vi "MainVI.vi"() -> ()   [LabVIEW 2020]
doc: "Main VI for Local Server on RPi and communication with cliend."
uses:
  <vilib>/MakerHub/LINX/Private/Type Defs/Peripherals/SPI/SPI Configuration.ctl
  <vilib>/MakerHub/LINX/Private/Type Defs/Peripherals/SPI/SPI Bit Order.ctl
  <vilib>/MakerHub/LINX/Private/Type Defs/Peripherals/SPI/SPI Mode.ctl
  Custom Ctls/Akcija.ctl
  Custom Ctls/States.ctl
  <vilib>/MediaMongrels Ltd/WebSockets/Sockets/VISA TCP Listener/VISA TCP Listener.lvclass
  <vilib>/MediaMongrels Ltd/WebSockets/WebSockets/WebSocket/WebSocket.lvclass
  <vilib>/MakerHub/LINX/Public/Peripherals/SPI/SPI CS Config.ctl
  <vilib>/MakerHub/LINX/Private/Type Defs/Peripherals/SPI/SPI CS Logic Level.ctl
  <vilib>/MediaMongrels Ltd/WebSockets/WebSockets/WebSocket Server/WebSocket Server.lvclass
  C:/Program Files (x86)/National Instruments/LabVIEW 2020/vi.lib/MediaMongrels Ltd/WebSockets/WebSockets/WebSocket/WebSocket.lvclass
  <vilib>/MakerHub/LINX/Public/Peripherals/SPI/SPI Write Read 1 Frame.vi
  <vilib>/MakerHub/LINX/Public/Peripherals/SPI/SPI Write Read N Frames.vi
  <vilib>/MakerHub/LINX/Private/Local IO/LinxSpiWriteRead.vi
  <vilib>/MakerHub/LINX/Public/Utilities/Check Channel.vi
  <vilib>/MakerHub/LINX/Private/Local IO/Handle Errors.vi
  <vilib>/MakerHub/LINX/Public/Utilities/Open Local.vi
  <vilib>/MakerHub/LINX/Private/Utilties/Generate Error.vi
  <vilib>/MakerHub/LINX/LMH-LINX.lvlib
panel:
  in  "Stop":bool
  out "String":string
  in  "Client Closed":string="The client VI closed the connection."
  in  "SPI Configuration":T1={"Clock Frequency"=1000000, "Bit Order"=enum."MSb First", "SPI Mode"=enum."Mode 0"}
  out "Output":u8[](array[numeric])
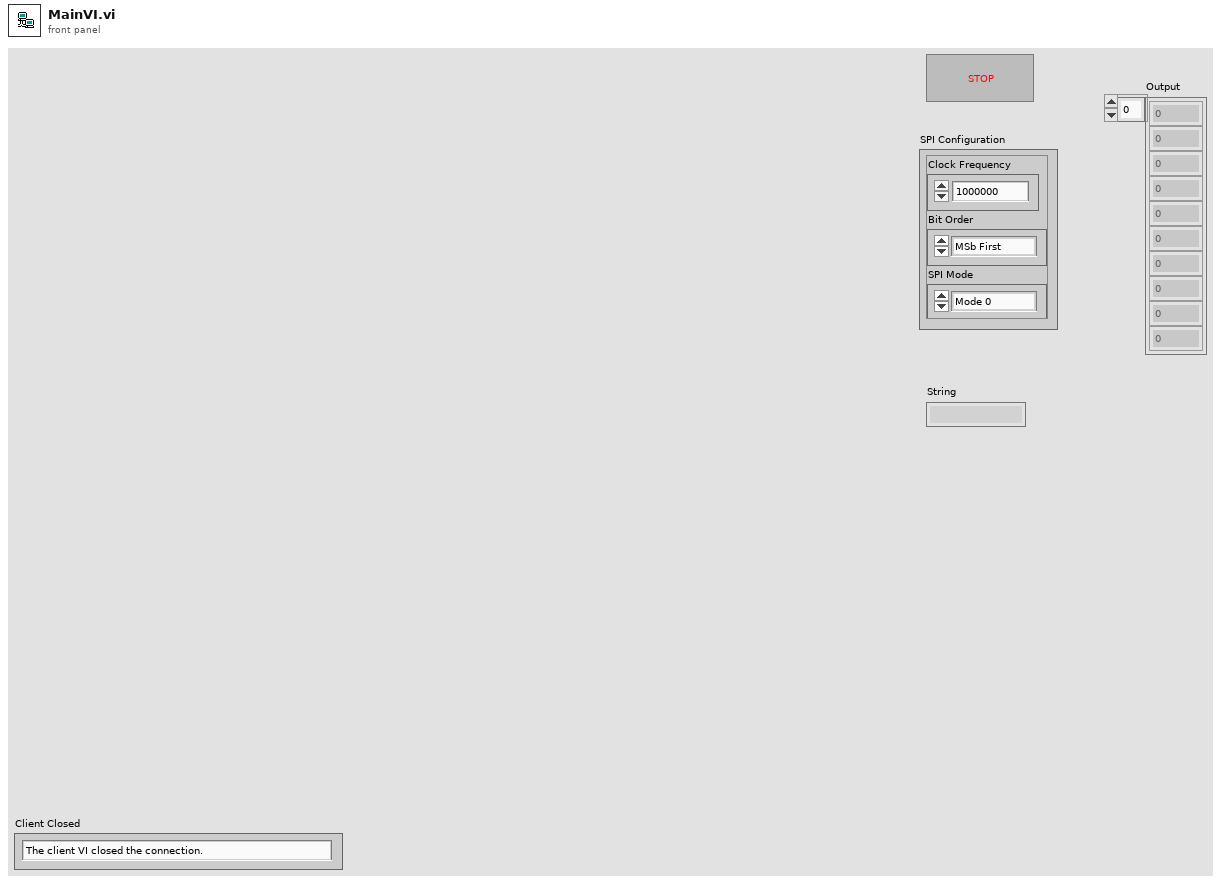
[diagram p1: front panel]
types:
  T1 = typedef "LMH-LINX.lvlib/SPI Configuration.ctl" = cluster{"Clock Frequency":u32, "Bit Order":T2, "SPI Mode":T3}
  T2 = typedef "LMH-LINX.lvlib/SPI Bit Order.ctl" = enum8{"LSb First", "MSb First"}
  T3 = typedef "LMH-LINX.lvlib/SPI Mode.ctl" = enum8{"Mode 0", "Mode 1", "Mode 2", "Mode 3"}
  T4 = typedef "States.ctl" = enum16{"Initialise", "Listen", "Read Data", "Close WebSocket", "Exit"}
  T5 = typedef "Akcija.ctl" = enum16{"Initialize", "Write", "Read", "Update"}
  T6 = typedef "LMH-LINX.lvlib/LINX Ref.ctl" = cluster{"IO":T7, "Interface":T8, "LINX Device Config":T9}
  T7 = typedef "LMH-LINX.lvlib/Platform.ctl" = enum16{"Remote", "Local"}
  T8 = typedef "LMH-LINX.lvlib/Interface.ctl" = enum16{"Serial", "TCP"}
  T9 = typedef "LMH-LINX.lvlib/Device.lvlib/LINX Device Config.ctl" = cluster{"Interface":T8, "COM Port":refnum<visa-resource-name>, "TCP Configuration":T10, "Device Family":u8, "Device ID":u8, "Device Name":string, "TCP Ref":refnum<k5>, "Channels":T11}
  T10 = typedef "LMH-LINX.lvlib/Device.lvlib/TCP Config.ctl" = cluster{"IP Address":string, "Port":u16}
  T11 = typedef "LMH-LINX.lvlib/Channels.ctl" = cluster{"DI":u8[], "DO":u8[], "AI":u8[], "AO":u8[], "PWM":u8[], "QE":u8[], "UART":u8[], "I2C 2":u8[], "SPI":u8[], "CAN":u8[], "Servo":u8[], "AI Ref (V)":dbl, "AI Resolution (Bits)":u8, "AO Ref (V)":dbl, "AO Resolution (Bits)":u8}
  T12 = typedef "LMH-LINX.lvlib/SPI CS Config.ctl" = cluster{"CS Channel":u8, "CS Logic Level":T13}
  T13 = typedef "LMH-LINX.lvlib/SPI CS Logic Level.ctl" = enum8{"Active Low", "Active High"}
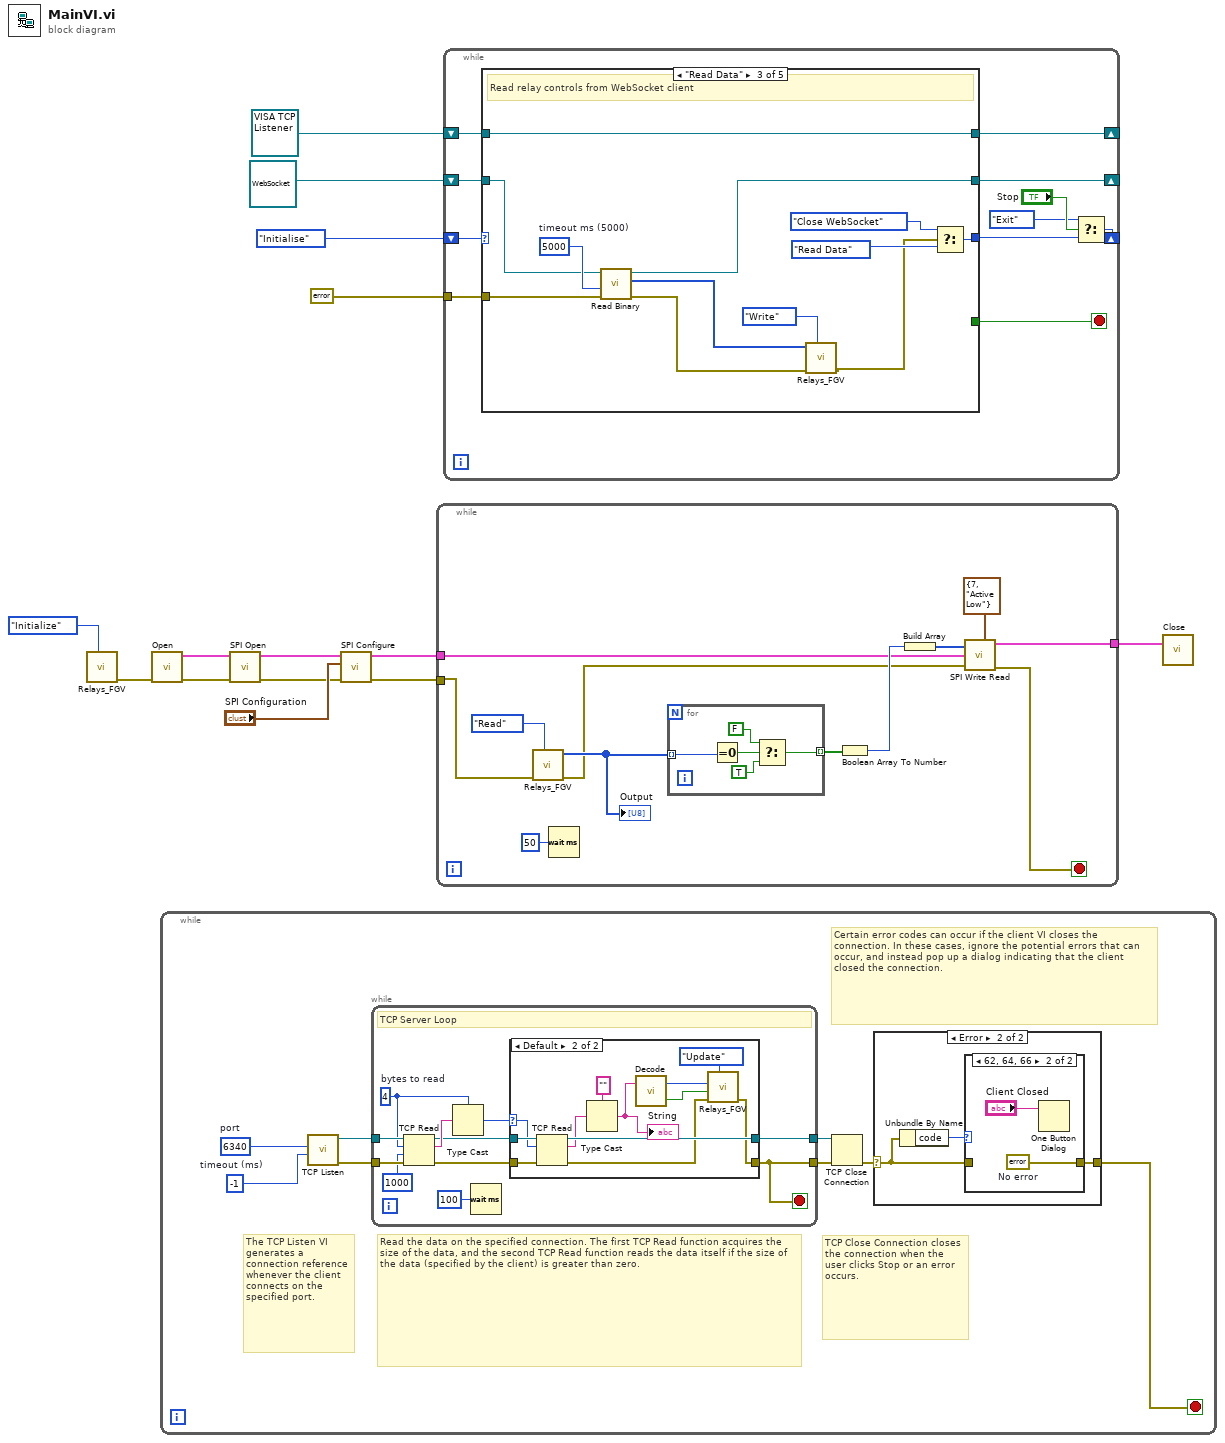
[diagram p0: block diagram]
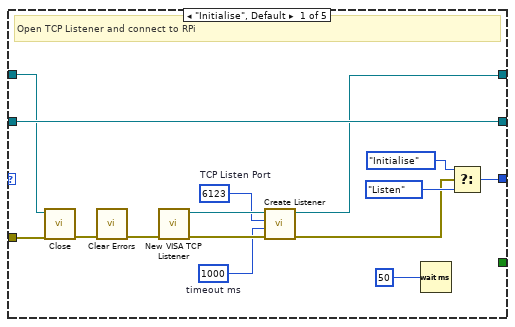
[diagram p2: hidden frame]
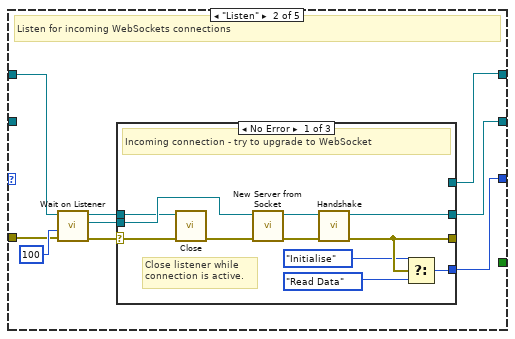
[diagram p3: hidden frame]
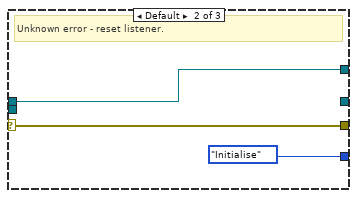
[diagram p4: hidden frame]
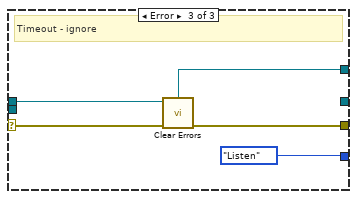
[diagram p5: hidden frame]
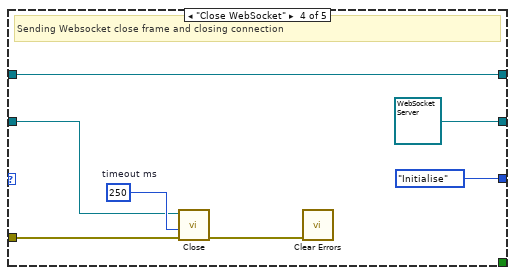
[diagram p6: hidden frame]
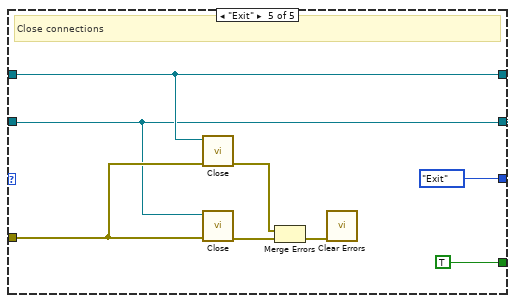
[diagram p7: hidden frame]
diagram:
  n1 = call "Relays_FGV.vi"("Akcija"=Akcija."Initialize") -> ("error out"=w8:errorcluster)  [unwired: 7 in, 1 out]
  n2 = call-poly <vilib>:"Open.vi"("Error In"=w8) -> ("Error Out"=w13:errorcluster, "LINX Resource"=w12:T6)  [unwired: 8 in, 1 out]
  n3 = while {
    stop <- w15 stop-if-true
    w21 = u16 6340  # port
    w22 = -1  # timeout (ms)
    # "TCP Close Connection closes the connection when the user clicks Stop or an error occurs."
    # "Certain error codes can occur if the client VI closes the connection. In these cases, ignore the potential errors that can occur, and instead pop up a dialog indicating that the client closed the connection."
    # "The TCP Listen VI generates a connection reference whenever the client connects on the specified port."
    # "Read the data on the specified connection. The first TCP Read function acquires the size of the data, and the second TCP Read function reads the data itself if the size of the data (specified by the client) is greater than zero."
    n4 = call <vilib>:"TCP Listen.vi"("timeout ms (wait forever: -1)"=w22, "port"=w21) -> ("error out"=w19:errorcluster, "connection ID"=w20:refnum<k5>)  [unwired: 5 in, 3 out]
    n5 = while {
      tunnel: w19 -> [w36]
      tunnel: w20 -> [w37]
      tunnel: [w33] -> w17
      tunnel: [w30] -> w16
      stop <- w30 stop-if-true
      w35 = 4  # bytes to read
      # "TCP Server Loop"
      n6 = TCP Read(connection ID=w37, bytes to read=w35, error in (no error)=w36, 9:1000 ("timeout ms (25000)")) -> (connection ID out=w39:refnum<k5>, data out=w40:string, error out=w38:errorcluster)  [unwired: 1 in]
      n7 = Type Cast(type=w35, x=w40) -> (*(type *) &x=w32:i32)
      n8 = Wait (ms)(milliseconds to wait=u32 100) -> ()  [unwired: 1 out]
      n9 = case shown="Default" w32 {
        selector: w32 -> [_ w50]
        tunnel: w39 -> [w42 w54]
        tunnel: w38 -> [w41 w53]
        tunnel: [w42 w52] -> w33
        tunnel: [w41 w43] -> w30
        frame ..0 {
          # "The server has not written any data"
        }
        frame Default {
          n10 = TCP Read(connection ID=w54, bytes to read=w50, error in (no error)=w53) -> (connection ID out=w52:refnum<k5>, data out=w51:string, error out=w44:errorcluster)  [unwired: 2 in]
          n11 = Type Cast(type="", x=w51) -> (*(type *) &x=w48:string)
          "String" <- w48
          n12 = call "Decode.vi"("String"=w48) -> ("ON/OFF"=w45:bool, "Relay Number"=w46:u8)  [unwired: 1 in]
          n13 = call "Relays_FGV.vi"("Akcija"=Akcija."Update", "error in (no error)"=w44, "ON/OFF"=w45, "Relay Number"=w46) -> ("error out"=w43:errorcluster)  [unwired: 4 in, 1 out]
        }
      }
    }
    n14 = TCP Close Connection(connection ID=w17, error in (no error)=w16) -> (error out=w18:errorcluster)  [unwired: 2 out]
    n15 = case shown="Error" w18 {
      selector: w18 -> [w23 w25]
      tunnel: [w23 w24] -> w15
      frame No Error {
      }
      frame Error {
        n16 = Unbundle By Name(w25) -> ("code"=w26:i32)
        n17 = case shown="62, 64, 66" w26 {
          tunnel: w25 -> [w27 _]
          tunnel: [w27 w29] -> w24
          frame Default {
          }
          frame 62, 64, 66 {
            w29 = errorcluster {"status"=FALSE, "code"=0, "source"=""}  # No error
            n18 = One Button Dialog(message="Client Closed") -> ()  [unwired: 1 in, 1 out]
          }
        }
      }
    }
  }
  n19 = call <vilib>:"SPI Open.vi"("Error In"=w13, "LINX Resource"=w12) -> ("Error Out"=w10:errorcluster, "LINX Resource"=w11:T6)  [unwired: 8 in]
  n20 = call <vilib>:"SPI Configure.vi"("Error In"=w10, "SPI Configuration"="SPI Configuration", "LINX Resource"=w11) -> ("Error Out"=w7:errorcluster, "LINX Resource"=w9:T6)  [unwired: 6 in, 1 out]
  n21 = while {
    tunnel: w9 -> [w60]
    tunnel: w7 -> [w61]
    tunnel: [w57] -> w6
    stop <- w58 stop-if-true
    n22 = call "Relays_FGV.vi"("Akcija"=Akcija."Read", "error in (no error)"=w61) -> ("error out"=w59:errorcluster, "Output"=w62:u8[])  [unwired: 6 in]
    "Output" <- w62
    n23 = Wait (ms)(milliseconds to wait=u32 50) -> ()  [unwired: 1 out]
    n24 = for {
      tunnel: [w68] -> w65 mode=indexing
      tunnel: w62 -> [w67] mode=indexing
      n25 = Equal To 0?(x=w67) -> (x = 0?=w71:bool)
      n26 = Select(t=FALSE, s=w71, f=TRUE) -> (s? t:f=w68:bool)
    }
    n27 = Boolean Array To Number(Boolean array=w65) -> (number=w64:u32)
    n28 = Build Array(w64) -> (w63:u32[])
    n29 = call-poly <vilib>:"SPI Write Read.vi"("CS Configuration"=T12 {"CS Channel"=7, "CS Logic Level"=enum."Active Low"}, "Error In"=w59, "Data"=w63, "LINX Resource"=w60) -> ("Error Out"=w58:errorcluster, "LINX Resource"=w57:T6)  [unwired: 4 in, 2 out]
  }
  n30 = while "Single Client WebSocket Server Demo" {
    shift-right: [w74] -> _
    shift-left: refnum<class "VISA TCP Listener.lvclass"> refnum ("VISA TCP Listener out") -> [w76]
    tunnel: errorcluster {"status"=FALSE, "code"=0, "source"=""} ("error constant") -> [w75]
    shift-right: [w81] -> _
    shift-left: States."Initialise" ("Enum") -> [w79]
    shift-right: [w77] -> _
    shift-left: refnum<class "WebSocket.lvclass"> refnum ("WebSocket out") -> [w78]
    stop <- w72 stop-if-true
    n31 = case shown="\"Read Data\"" w79 {
      tunnel: [w90 w99 w135 refnum<class "WebSocket Server.lvclass"> refnum ("WebSocket out") w145] -> w77
      tunnel: w78 -> [w90 _ w133 w140 w145]
      tunnel: w76 -> [w89 w101 w134 w138 w146]
      tunnel: w75 -> [w88 w102 w132 w141 w148]
      tunnel: [w87 w98 w134 w138 w146] -> w74
      tunnel: [w84 w100 w129 States."Initialise" ("Enum") States."Exit" ("Enum")] -> w73
      tunnel: [_ _ _ _ TRUE] -> w72
      frame "Initialise", Default {
        w94 = 1000  # timeout ms
        w95 = u16 6123  # TCP Listen Port
        # "Open TCP Listener and connect to RPi"
        n32 = call-dynamic <vilib>:"Close.vi"("error in (no error)"=w88, "VISA TCP Listener in"=w89) -> ("error out"=w92:errorcluster)  [unwired: 9 in]
        n33 = call <vilib>:"Clear Errors.vi"("error in (no error)"=w92) -> ("error out"=w91:errorcluster)  [unwired: 5 in, 1 out]
        n34 = call <vilib>:"New VISA TCP Listener.vi"("error in (no error)"=w91) -> ("error out"=w96:errorcluster, "VISA TCP Listener out"=w97:refnum<class "VISA TCP Listener.lvclass">)  [unwired: 9 in]
        n35 = call-dynamic "Create Listener.vi"("error in (no error)"=w96, "timeout ms (5000)"=w94, "Port"=w95, "VISA TCP Listener in"=w97) -> ("error out"=w83:errorcluster, "VISA TCP Listener out"=w87:refnum<class "VISA TCP Listener.lvclass">)  [unwired: 6 in]
        n36 = Wait (ms)(milliseconds to wait=u32 50) -> ()  [unwired: 1 out]
        n37 = Select(t=States."Initialise" ("Enum"), s=w83, f=States."Listen" ("Enum")) -> (s? t:f=w84:T4)
      }
      frame "Listen" {
        # "Listen for incoming WebSockets connections"
        n38 = call-dynamic "Wait on Listener.vi"("error in (no error)"=w102, "timeout ms (5000)"=100, "VISA TCP Listener in"=w101) -> ("error out"=w105:errorcluster, "Socket out"=w106:refnum<class "Socket.lvclass">, "VISA TCP Listener out"=w104:refnum<class "VISA TCP Listener.lvclass">)  [unwired: 6 in]
        n39 = case shown="No Error" w105 {
          selector: w105 -> [w113 w120 w124]
          tunnel: w106 -> [w115 _ _]
          tunnel: w104 -> [w112 w119 w123]
          tunnel: [w111 _ _] -> w99
          tunnel: [w110 w120 w122] -> _
          tunnel: [_ w119 w123] -> w98
          tunnel: [w107 States."Initialise" ("Enum") States."Listen" ("Enum")] -> w100
          frame No Error {
            # "Close listener while connection is active."
            # "Incoming connection - try to upgrade to WebSocket"
            n40 = call-dynamic <vilib>:"Close.vi"("error in (no error)"=w113, "VISA TCP Listener in"=w112) -> ("error out"=w114:errorcluster)  [unwired: 9 in]
            n41 = call <vilib>:"New Server from Socket.vi"("error in (no error)"=w114, "Socket"=w115) -> ("error out"=w116:errorcluster, "WebSocket Server out"=w117:refnum<class "WebSocket Server.lvclass">)  [unwired: 8 in]
            n42 = call-dynamic "Handshake.vi"("error in (no error)"=w116, "WebSocket Connection in"=w117) -> ("error out"=w110:errorcluster, "WebSocket Connection out"=w111:refnum<class "WebSocket Server.lvclass">)  [unwired: 8 in]
            n43 = Select(t=States."Initialise" ("Enum"), s=w110, f=States."Read Data" ("Enum")) -> (s? t:f=w107:T4)
          }
          frame Default {
            # "Unknown error - reset listener."
          }
          frame Error {
            # "Timeout - ignore"
            n44 = call <vilib>:"Clear Errors.vi"("error in (no error)"=w124) -> ("error out"=w122:errorcluster)  [unwired: 5 in, 1 out]
          }
        }
      }
      frame "Read Data" {
        w136 = 5000  # timeout ms (5000)
        # "Read relay controls from WebSocket client"
        n45 = call-dynamic "Read Binary.vi"("error in (no error)"=w132, "timeout ms (5000)"=w136, "WebSocket in"=w133) -> ("error out"=w127:errorcluster, "Data"=w128:u8[], "WebSocket out"=w135:refnum<class "WebSocket.lvclass">)  [unwired: 6 in]
        n46 = call "Relays_FGV.vi"("Akcija"=Akcija."Write", "error in (no error)"=w127, "Input"=w128) -> ("error out"=w126:errorcluster)  [unwired: 5 in, 1 out]
        n47 = Select(t=States."Close WebSocket" ("Enum"), s=w126, f=States."Read Data" ("Enum")) -> (s? t:f=w129:T4)
      }
      frame "Close WebSocket" {
        w142 = 250  # timeout ms
        # "Sending Websocket close frame and closing connection"
        n48 = call-dynamic <vilib>:"Close.vi"("error in (no error)"=w141, "timeout ms (5000)"=w142, "WebSocket in"=w140) -> ("error out"=w143:errorcluster)  [unwired: 8 in]
        n49 = call <vilib>:"Clear Errors.vi"("error in (no error)"=w143) -> ()  [unwired: 5 in, 2 out]
      }
      frame "Exit" {
        # "Close connections"
        n50 = call-dynamic <vilib>:"Close.vi"("error in (no error)"=w148, "VISA TCP Listener in"=w146) -> ("error out"=w150:errorcluster)  [unwired: 9 in]
        n51 = call-dynamic <vilib>:"Close.vi"("error in (no error)"=w148, "WebSocket in"=w145) -> ("error out"=w149:errorcluster)  [unwired: 9 in]
        n52 = Merge Errors(w150, w149) -> (w151:errorcluster)
        n53 = call <vilib>:"Clear Errors.vi"("error in (no error)"=w151) -> ()  [unwired: 5 in, 2 out]
      }
    }
    n54 = Select(t=States."Exit" ("Enum"), s="Stop", f=w73) -> (s? t:f=w81:T4)
  }
  n55 = call <vilib>:"Close.vi"("LINX Resource"=w6) -> ()  [unwired: 10 in, 1 out]
